vi "top_GameMode.vi"() -> ()   [LabVIEW 2014]
uses:
  <vilib>/sound2/lvsound2.llb/Sound Data Format.ctl
  <vilib>/sound2/lvsound2.llb/Sound Output Set Volume (Single).vi
  <vilib>/Utility/inputDevices.llb/keyboardAcquire.vi
  <vilib>/sound2/lvsound2.llb/Sound Output Write (DBL Single).vi
  <vilib>/Utility/inputDevices.llb/closeKeyboard.vi
  <vilib>/measure/NI_MABase.lvlib
panel:
  in  "stop":bool
  out "Your Score":dbl
  out "score":i32
  out "appended array 2":u32[](array[numeric])
  out "24":bool
  out "23":bool
  out "22":bool
  out "21":bool
  out "20":bool
  out "19":bool
  out "18":bool
  out "17":bool
  out "16":bool
  out "15":bool caption="Boolean 15"
  out "14":bool caption="Boolean 14"
  out "13":bool caption="Boolean 13"
  out "12":bool caption="Boolean 12"
  out "11":bool
  out "10":bool
  out "9":bool
  out "8":bool
  out "7":bool
  out "6":bool
  out "5":bool
  out "4":bool
  in  "Volume":dbl=70.0
  in  "Mode":enum16{"keypad", "button"}(ring)
  in  "Cluster":T1
  out "element 2":T2(ring)
  out "press time":u32[](array[numeric])
  out "String":string="3"
  out "3":bool
  out "2":bool
  out "1":bool
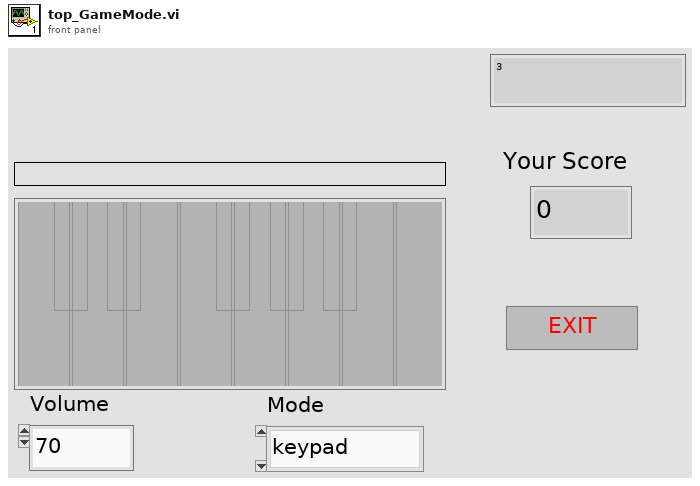
[diagram p1: front panel]
types:
  T1 = cluster{"c 2":bool, "c 3":bool, "c 4":bool, "c 5":bool, "c 6":bool, "c 7":bool, "c 8":bool, "c 9":bool, "c":bool, "c 10":bool, "c 11":bool, "c 12":bool, "c 13":bool}
  T2 = enum16{"0", "1", "2", "3", "4", "5", "6", "7", "8", "9", "A", "B", "C", "D", "E", "F", "G", "H", "I", "J", "K", "L", "M", "N", "O", "P", "Q", "R", "S", "T", "U", "V", "W", "X", "Y", "Z", "F1", "F2", "F3", "F4", "F5", "F6", "F7", "F8", "F9", "F10", "F11", "F12", "F13", "F14", "F15", "ADD", "BACK", "BACKSLASH", "CAPITAL", "COMMA", "DECIMAL", "DELETE", "DIVIDE", "DOWN", "END", "EQUALS", "ESCAPE", "GRAVE (`)", "HOME", "INSERT", "LBRACKET", "LCONTROL", "LEFT", "L ALT", "LSHIFT", "LWIN", "MINUS", "MULTIPLY", "NEXT", "NUMLOCK", "NUMPAD_0", "NUMPAD_1", "NUMPAD_2", "NUMPAD_3", "NUMPAD_4", "NUMPAD_5", "NUMPAD_6", "NUMPAD_7", "NUMPAD_8", "NUMPAD_9", "PAUSE", "PERIOD", "PRIOR (PG UP)", "RBRACKET", "RCONTROL", "RETURN", "RIGHT", "R ALT", "RSHIFT", "RWIN", "SCROLL", "SEMICOLON", "SLASH", "SPACE", "SUBTRACT", "TAB", "UP", "ENTER (num pad)", "' (quote)"}
  T3 = typedef "Sound Data Format.ctl" = cluster{"sample rate (S/s)":dbl, "number of channels":i32, "bits per sample":i32}
  T4 = typedef "Sound Output Task ID.ctl" = u32
  T5 = cluster{"sample rate (S/s)":dbl, "number of samples/ch":i32}
  T6 = enum16{"0", "1", "2", "3", "4", "5", "6", "7", "8", "9", "A", "B", "C", "D", "E", "F", "G", "H", "I", "J", "K", "L", "M", "N", "O", "P", "Q", "R", "S", "T", "U", "V", "W", "X", "Y", "Z", "F1", "F2", "F3", "F4", "F5", "F6", "F7", "F8", "F9", "F10", "F11", "F12", "F13", "F14", "F15", "ADD", "BACK", "BACKSLASH", "CAPITAL", "COMMA", "DECIMAL", "DELETE", "DIVIDE", "DOWN", "END", "EQUALS", "ESCAPE", "GRAVE (`)", "HOME", "INSERT", "LBRACKET", "LCONTROL", "LEFT", "L ALT", "LSHIFT", "LWIN", "MINUS", "MULTIPLY", "NEXT", "NUMLOCK", "NUMPAD_0", "NUMPAD_1", "NUMPAD_2", "NUMPAD_3", "NUMPAD_4", "NUMPAD_5", "NUMPAD_6", "NUMPAD_7", "NUMPAD_8", "NUMPAD_9", "PAUSE", "PERIOD", "PRIOR (PG UP)", "RBRACKET", "RCONTROL", "RETURN", "RIGHT", "R ALT", "RSHIFT", "RWIN", "SCROLL", "SEMICOLON", "SLASH", "SPACE", "SUBTRACT", "TAB", "UP", "ENTER (num pad)", "' (quote)"}[]
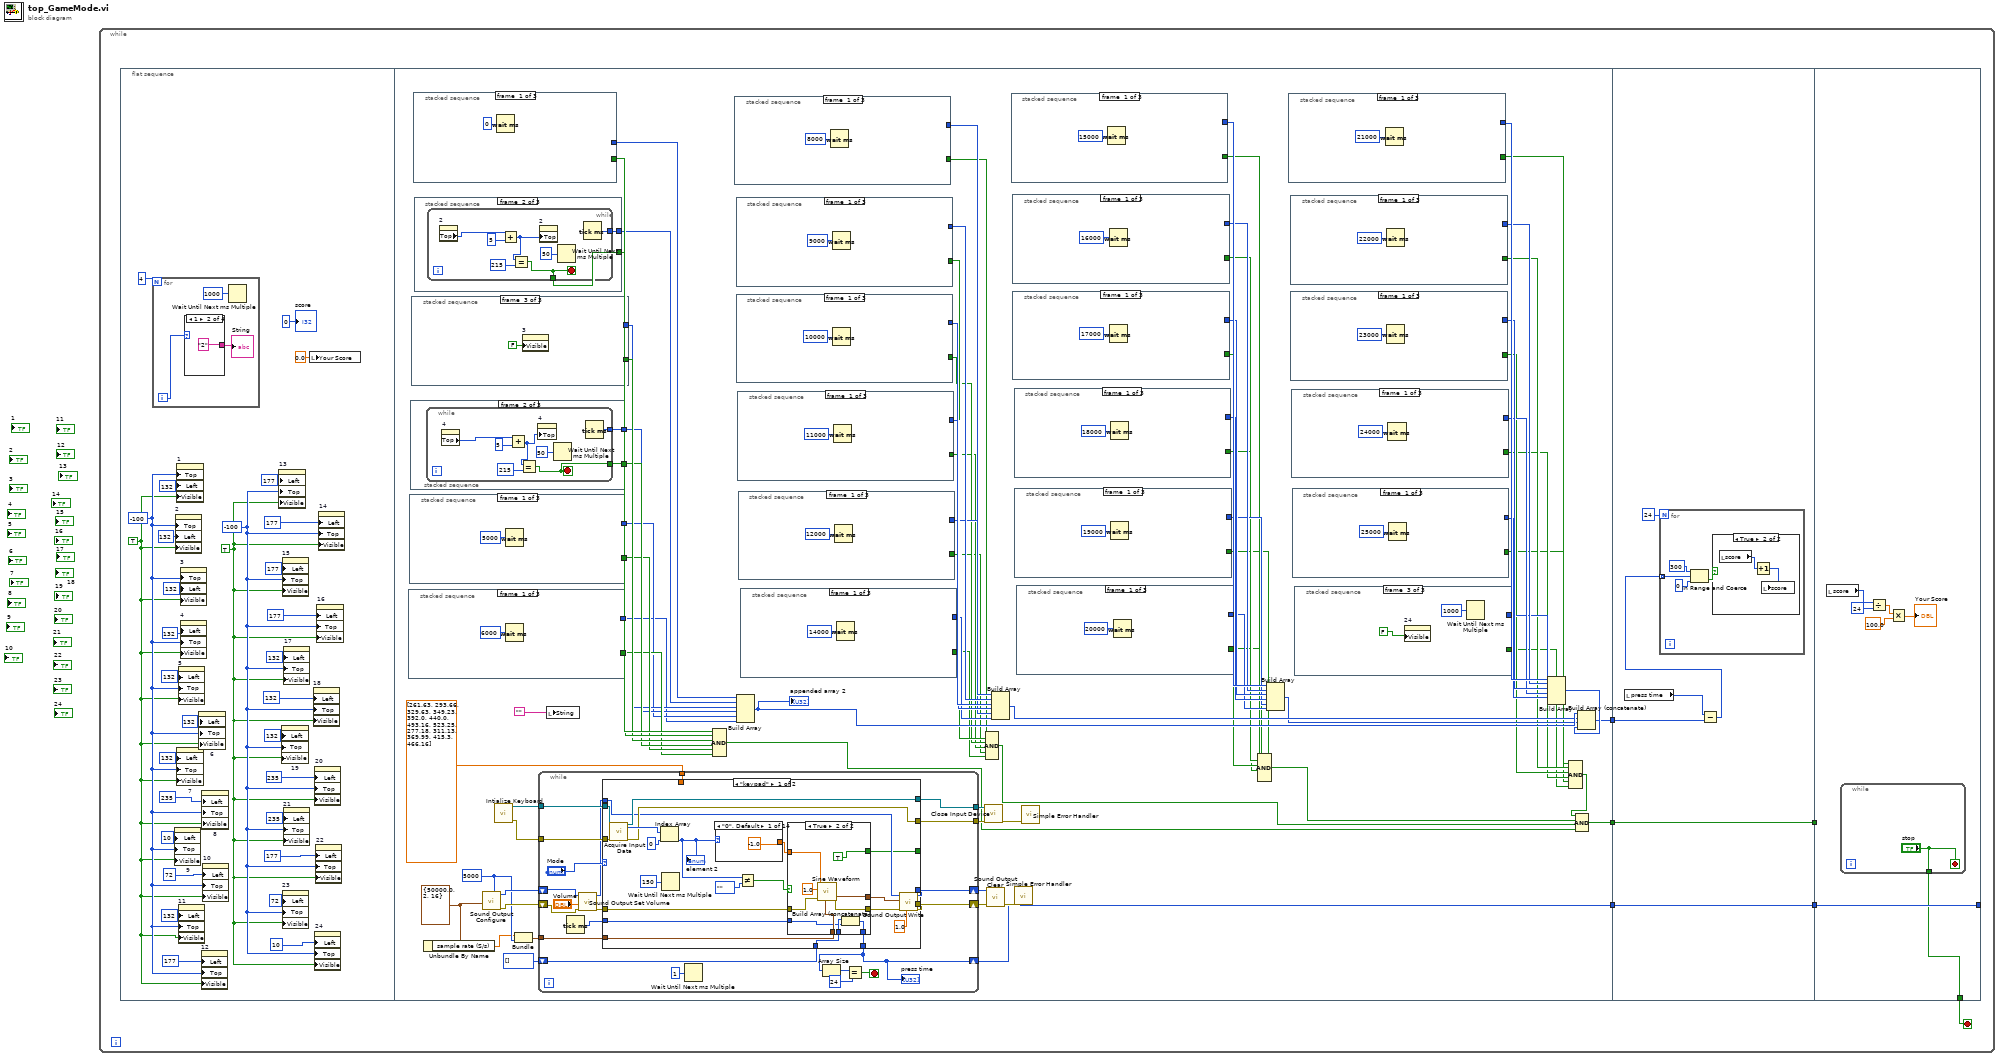
[diagram p0: block diagram]
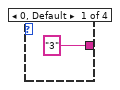
[diagram p2: hidden frame]
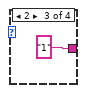
[diagram p3: hidden frame]
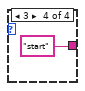
[diagram p4: hidden frame]
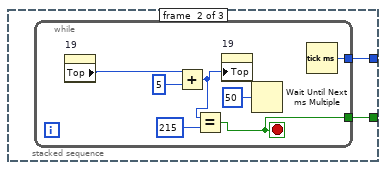
[diagram p5: hidden frame]
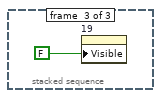
[diagram p6: hidden frame]
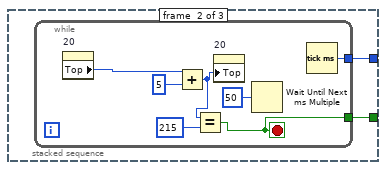
[diagram p7: hidden frame]
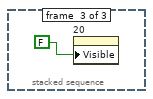
[diagram p8: hidden frame]
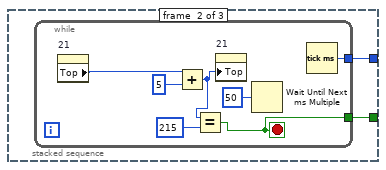
[diagram p9: hidden frame]
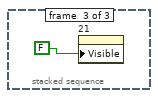
[diagram p10: hidden frame]
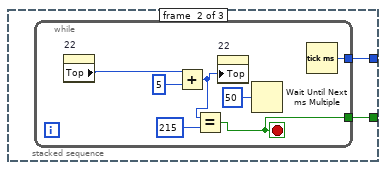
[diagram p11: hidden frame]
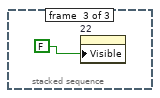
[diagram p12: hidden frame]
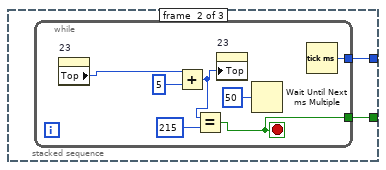
[diagram p13: hidden frame]
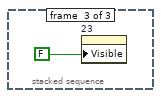
[diagram p14: hidden frame]
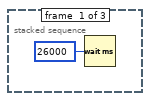
[diagram p15: hidden frame]
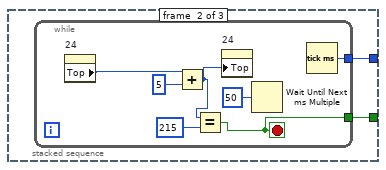
[diagram p16: hidden frame]
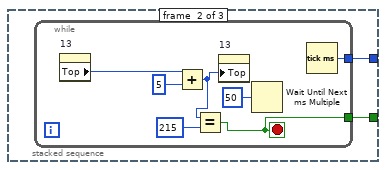
[diagram p17: hidden frame]
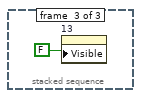
[diagram p18: hidden frame]
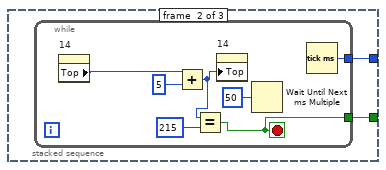
[diagram p19: hidden frame]
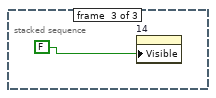
[diagram p20: hidden frame]
diagram:
  n1 = while {
    stop <- w1 stop-if-true
    n2 = flat-sequence {
      tunnel: [w104] -> w6
      tunnel: [w47] -> w5
      tunnel: [w46] -> w2
      tunnel: w6 -> [w496]
      tunnel: w5 -> [w495]
      tunnel: [w496] -> w4
      tunnel: [w491] -> w3
      tunnel: w2 -> [w491]
      tunnel: [w509] -> _
      tunnel: w4 -> [w509]
      tunnel: w3 -> [_]
      tunnel: [w503] -> w1
      frame #0 {
        w9 = TRUE
        w10 = TRUE
        w32 = -100
        w33 = -100
        n3 = for {
          N: 4 -> [_]
          i -> [w40]
          n4 = case shown="1" w40 {
            tunnel: ["3" "2" "1" "start"] -> w38
            frame 0, Default {
            }
            frame 1 {
            }
            frame 2 {
            }
            frame 3 {
            }
          }
          "String" <- w38
          n5 = Wait Until Next ms Multiple(millisecond multiple=u32 1000) -> ()  [unwired: 1 out]
        }
        n6 = property on="9" class="Bool (strict)"("Left"=10 ("Position:Left"), "Top"=w33, "Visible"=w10) -> ()  [unwired: 2 in, 2 out]
        n7 = property on="2" class="Bool (strict)"("Top"=w33, "Left"=132 ("Position:Left"), "Visible"=w10) -> ()  [unwired: 2 in, 2 out]
        n8 = property on="1" class="Bool (strict)"("Top"=w33, "Left"=132 ("Position:Left"), "Visible"=w10) -> ()  [unwired: 2 in, 2 out]
        n9 = property on="7" class="Bool (strict)"("Left"=132 ("Position:Left"), "Top"=w33, "Visible"=w10) -> ()  [unwired: 2 in, 2 out]
        n10 = property on="5" class="Bool (strict)"("Left"=132 ("Position:Left"), "Top"=w33, "Visible"=w10) -> ()  [unwired: 2 in, 2 out]
        n11 = property on="11" class="Bool (strict)"("Left"=132 ("Position:Left"), "Top"=w33, "Visible"=w10) -> ()  [unwired: 2 in, 2 out]
        n12 = property on="3" class="Bool (strict)"("Top"=w33, "Left"=132 ("Position:Left"), "Visible"=w10) -> ()  [unwired: 2 in, 2 out]
        n13 = property on="4" class="Bool (strict)"("Left"=132 ("Position:Left"), "Top"=w33, "Visible"=w10) -> ()  [unwired: 2 in, 2 out]
        n14 = property on="6" class="Bool (strict)"("Left"=132 ("Position:Left"), "Top"=w33, "Visible"=w10) -> ()  [unwired: 2 in, 2 out]
        n15 = property on="12" class="Bool (strict)"("Left"=177 ("Position:Left"), "Top"=w33, "Visible"=w10) -> ()  [unwired: 2 in, 2 out]
        n16 = property on="8" class="Bool (strict)"("Left"=235 ("Position:Left"), "Top"=w33, "Visible"=w10) -> ()  [unwired: 2 in, 2 out]
        n17 = property on="10" class="Bool (strict)"("Left"=72 ("Position:Left"), "Top"=w33, "Visible"=w10) -> ()  [unwired: 2 in, 2 out]
        n18 = property on="13" class="Bool (strict)"("Left"=177 ("Position:Left"), "Top"=w32, "Visible"=w9) -> ()  [unwired: 2 in, 2 out]
        n19 = property on="19" class="Bool (strict)"("Left"=132 ("Position:Left"), "Top"=w32, "Visible"=w9) -> ()  [unwired: 2 in, 2 out]
        n20 = property on="15" class="Bool (strict)"("Left"=177 ("Position:Left"), "Top"=w32, "Visible"=w9) -> ()  [unwired: 2 in, 2 out]
        n21 = property on="23" class="Bool (strict)"("Left"=72 ("Position:Left"), "Top"=w32, "Visible"=w9) -> ()  [unwired: 2 in, 2 out]
        n22 = property on="17" class="Bool (strict)"("Left"=132 ("Position:Left"), "Top"=w32, "Visible"=w9) -> ()  [unwired: 2 in, 2 out]
        n23 = property on="21" class="Bool (strict)"("Left"=235 ("Position:Left"), "Top"=w32, "Visible"=w9) -> ()  [unwired: 2 in, 2 out]
        n24 = local write "Your Score"(0.0 ("your score")) -> ()
        n25 = property on="18" class="Bool (strict)"("Left"=132 ("Position:Left"), "Top"=w32, "Visible"=w9) -> ()  [unwired: 2 in, 2 out]
        n26 = property on="20" class="Bool (strict)"("Left"=235 ("Position:Left"), "Top"=w32, "Visible"=w9) -> ()  [unwired: 2 in, 2 out]
        n27 = property on="24" class="Bool (strict)"("Left"=10 ("Position:Left"), "Top"=w32, "Visible"=w9) -> ()  [unwired: 2 in, 2 out]
        n28 = property on="22" class="Bool (strict)"("Left"=177 ("Position:Left"), "Top"=w32, "Visible"=w9) -> ()  [unwired: 2 in, 2 out]
        n29 = property on="16" class="Bool (strict)"("Left"=177 ("Position:Left"), "Top"=w32, "Visible"=w9) -> ()  [unwired: 2 in, 2 out]
        n30 = property on="14" class="Bool (strict)"("Left"=177 ("Position:Left"), "Top"=w32, "Visible"=w9) -> ()  [unwired: 2 in, 2 out]
        "score" <- 0
      }
      frame #1 {
        w117 = 5000 ("number of samples/ch")
        w118 = T3 {"sample rate (S/s)"=50000.0, "number of channels"=2, "bits per sample"=16} ("sound format")
        n31 = stacked-sequence {
          tunnel: [_ w333 _] -> w98
          tunnel: [_ w332 _] -> w92
          frame #0 {
            n32 = Wait (ms)(milliseconds to wait=u32 6000) -> ()  [unwired: 1 out]
          }
          frame #1 {
            n33 = while {
              tunnel: [w337] -> w333
              tunnel: [w336] -> w332
              stop <- w337 stop-if-true
              n34 = property on="6" class="Bool (strict)"() -> ("Top"=w334:i32)  [unwired: 2 in, 2 out]
              n35 = Add(x=w334, y=5) -> (x+y=w335:i32)
              n36 = Equal?(x=w335, y=215) -> (x = y?=w337:bool)
              n37 = property on="6" class="Bool (strict)"("Top"=w335) -> ()  [unwired: 2 in, 2 out]
              n38 = Wait Until Next ms Multiple(millisecond multiple=u32 50) -> ()  [unwired: 1 out]
              n39 = Tick Count (ms)() -> (millisecond timer value=w336:u32)
            }
          }
          frame #2 {
            n40 = property on="6" class="Bool (strict)"("Visible"=FALSE) -> ()  [unwired: 2 in, 2 out]
          }
        }
        n41 = stacked-sequence {
          tunnel: [_ w344 _] -> w99
          tunnel: [_ w343 _] -> w93
          frame #0 {
            n42 = Wait (ms)(milliseconds to wait=u32 5000) -> ()  [unwired: 1 out]
          }
          frame #1 {
            n43 = while {
              tunnel: [w348] -> w344
              tunnel: [w347] -> w343
              stop <- w348 stop-if-true
              n44 = property on="5" class="Bool (strict)"() -> ("Top"=w345:i32)  [unwired: 2 in, 2 out]
              n45 = Add(x=w345, y=5) -> (x+y=w346:i32)
              n46 = Equal?(x=w346, y=215) -> (x = y?=w348:bool)
              n47 = property on="5" class="Bool (strict)"("Top"=w346) -> ()  [unwired: 2 in, 2 out]
              n48 = Wait Until Next ms Multiple(millisecond multiple=u32 50) -> ()  [unwired: 1 out]
              n49 = Tick Count (ms)() -> (millisecond timer value=w347:u32)
            }
          }
          frame #2 {
            n50 = property on="5" class="Bool (strict)"("Visible"=FALSE) -> ()  [unwired: 2 in, 2 out]
          }
        }
        n51 = stacked-sequence {
          tunnel: [_ w355 _] -> w100
          tunnel: [_ w354 _] -> w94
          frame #0 {
            n52 = Wait (ms)(milliseconds to wait=u32 4000) -> ()  [unwired: 1 out]
          }
          frame #1 {
            n53 = while {
              tunnel: [w359] -> w355
              tunnel: [w358] -> w354
              stop <- w359 stop-if-true
              n54 = property on="4" class="Bool (strict)"() -> ("Top"=w356:i32)  [unwired: 2 in, 2 out]
              n55 = Add(x=w356, y=5) -> (x+y=w357:i32)
              n56 = Equal?(x=w357, y=215) -> (x = y?=w359:bool)
              n57 = property on="4" class="Bool (strict)"("Top"=w357) -> ()  [unwired: 2 in, 2 out]
              n58 = Wait Until Next ms Multiple(millisecond multiple=u32 50) -> ()  [unwired: 1 out]
              n59 = Tick Count (ms)() -> (millisecond timer value=w358:u32)
            }
          }
          frame #2 {
            n60 = property on="4" class="Bool (strict)"("Visible"=FALSE) -> ()  [unwired: 2 in, 2 out]
          }
        }
        n61 = stacked-sequence {
          tunnel: [_ w471 _] -> w101
          tunnel: [_ w470 _] -> w95
          frame #0 {
            n62 = Wait (ms)(milliseconds to wait=u32 2000) -> ()  [unwired: 1 out]
          }
          frame #1 {
            n63 = while {
              tunnel: [w474] -> w471
              tunnel: [w472] -> w470
              stop <- w474 stop-if-true
              n64 = property on="3" class="Bool (strict)"() -> ("Top"=w475:i32)  [unwired: 2 in, 2 out]
              n65 = Add(x=w475, y=5) -> (x+y=w473:i32)
              n66 = Equal?(x=w473, y=215) -> (x = y?=w474:bool)
              n67 = property on="3" class="Bool (strict)"("Top"=w473) -> ()  [unwired: 2 in, 2 out]
              n68 = Wait Until Next ms Multiple(millisecond multiple=u32 50) -> ()  [unwired: 1 out]
              n69 = Tick Count (ms)() -> (millisecond timer value=w472:u32)
            }
          }
          frame #2 {
            n70 = property on="3" class="Bool (strict)"("Visible"=FALSE) -> ()  [unwired: 2 in, 2 out]
          }
        }
        n71 = stacked-sequence {
          tunnel: [_ w322 _] -> w103
          tunnel: [_ w321 _] -> w97
          frame #0 {
            n72 = Wait (ms)(milliseconds to wait=u32 0) -> ()  [unwired: 1 out]
          }
          frame #1 {
            n73 = while {
              tunnel: [w324] -> w322
              tunnel: [w323] -> w321
              stop <- w324 stop-if-true
              n74 = property on="1" class="Bool (strict)"() -> ("Top"=w328:i32)  [unwired: 2 in, 2 out]
              n75 = Add(x=w328, y=5) -> (x+y=w326:i32)
              n76 = Equal?(x=w326, y=215) -> (x = y?=w324:bool)
              n77 = property on="1" class="Bool (strict)"("Top"=w326) -> ()  [unwired: 2 in, 2 out]
              n78 = Wait Until Next ms Multiple(millisecond multiple=u32 50) -> ()  [unwired: 1 out]
              n79 = Tick Count (ms)() -> (millisecond timer value=w323:u32)
            }
          }
          frame #2 {
            n80 = property on="1" class="Bool (strict)"("Visible"=FALSE) -> ()  [unwired: 2 in, 2 out]
          }
        }
        n81 = stacked-sequence {
          tunnel: [_ w482 _] -> w102
          tunnel: [_ w481 _] -> w96
          frame #0 {
            n82 = Wait (ms)(milliseconds to wait=u32 1000) -> ()  [unwired: 1 out]
          }
          frame #1 {
            n83 = while {
              tunnel: [w484] -> w482
              tunnel: [w483] -> w481
              stop <- w484 stop-if-true
              n84 = property on="2" class="Bool (strict)"() -> ("Top"=w487:i32)  [unwired: 2 in, 2 out]
              n85 = Add(x=w487, y=5) -> (x+y=w485:i32)
              n86 = Equal?(x=w485, y=215) -> (x = y?=w484:bool)
              n87 = property on="2" class="Bool (strict)"("Top"=w485) -> ()  [unwired: 2 in, 2 out]
              n88 = Wait Until Next ms Multiple(millisecond multiple=u32 50) -> ()  [unwired: 1 out]
              n89 = Tick Count (ms)() -> (millisecond timer value=w483:u32)
            }
          }
          frame #2 {
            n90 = property on="2" class="Bool (strict)"("Visible"=FALSE) -> ()  [unwired: 2 in, 2 out]
          }
        }
        n91 = Unbundle By Name(w118) -> ("sample rate (S/s)"=w116:dbl)
        n92 = call <vilib>:"Sound Output Configure.vi"("number of samples/ch"=w117, "sound format"=w118) -> ("error out"=w119:errorcluster, "task ID"=w120:T4)  [unwired: 8 in]
        n93 = call <vilib>:"Intialize Keyboard.vi"() -> ("error out"=w109:errorcluster, "device ID"=w108:refnum<k1>)  [unwired: 10 in]
        n94 = Bundle("sample rate (S/s)"=w116, "number of samples/ch"=w117) -> (w115:T5)  [unwired: 1 in]
        n95 = while {
          tunnel: w115 -> [w381]
          tunnel: dbl[] [261.63, 293.66, 329.63, 349.23, 392.0, 440.0, 493.16, 523.25, 277.18, 311.13, 369.99, 415.3, 466.16] -> [w377]
          shift-right: [w380] -> w114
          shift-left: w120 -> [w383]
          shift-right: [w379] -> w113
          shift-left: w119 -> [w378]
          tunnel: w109 -> [w374]
          tunnel: w108 -> [w373]
          tunnel: [w372] -> w107
          tunnel: [w371] -> w106
          shift-right: [w367] -> w104
          shift-left: u32[] [] -> [w369]
          stop <- w364 stop-if-true
          n96 = Tick Count (ms)() -> (millisecond timer value=w368:u32)
          n97 = call-poly <vilib>:"Sound Output Set Volume.vi"("error in (no error)"=w378, "volume"="Volume", "task ID"=w383) -> ("error out"=w382:errorcluster, "task ID out"=w370:T4)  [unwired: 7 in]
          n98 = case shown="\"keypad\"" "Mode" {
            tunnel: w382 -> [w394 w453]
            tunnel: w381 -> [w393 w450]
            tunnel: w370 -> [w392 w449]
            tunnel: [w391 w448] -> w380
            tunnel: [w390 w447] -> w379
            tunnel: w377 -> [_ w446]
            tunnel: w374 -> [w398 _]
            tunnel: w373 -> [w397 _]
            tunnel: [w396 _] -> w372
            tunnel: [w395 _] -> w371
            tunnel: [w389 w438] -> _
            tunnel: w369 -> [w388 w437]
            tunnel: [w387 w436] -> w367
            tunnel: w368 -> [w386 w435]
            frame "keypad" {
              n99 = call-poly <vilib>:"Acquire Input Data.vi"("device ID"=w397, "error in (no error)"=w398) -> ("device ID"=w396:refnum<k1>, "keys pressed"=w403:T6, "error out"=w395:errorcluster)  [unwired: 15 in]
              n100 = Index Array(array=w403, index=0) -> (element=w407:T2)
              "element 2" <- w407
              n101 = Wait Until Next ms Multiple(millisecond multiple=u32 150) -> ()  [unwired: 1 out]
              n102 = case shown="\"0\", Default" w407 {
                tunnel: [-1.0 261.63 277.18 293.66 311.13 329.63 349.23 369.99 392 415.3 440 466.16 493.88 523.25] -> w402
                frame "0", Default {
                }
                frame "S" {
                }
                frame "E" {
                }
                frame "D" {
                }
                frame "R" {
                }
                frame "F" {
                }
                frame "G" {
                }
                frame "Y" {
                }
                frame "H" {
                }
                frame "U" {
                }
                frame "J" {
                }
                frame "I" {
                }
                frame "K" {
                }
                frame "L" {
                }
              }
              n103 = Not Equal?(x=w407, y=enum16{""}."") -> (x != y?=w406:bool)
              n104 = case shown="True" w406 {
                tunnel: w394 -> [w410 w419]
                tunnel: [_ w418] -> w399
                tunnel: [w410 w417] -> w400
                tunnel: w393 -> [_ w416]
                tunnel: w402 -> [_ w415]
                tunnel: [FALSE TRUE] -> w389
                tunnel: w388 -> [w408 w413]
                tunnel: [w408 w412] -> w387
                tunnel: w386 -> [_ w411]
                frame False {
                }
                frame True {
                  n105 = call <vilib>:"Sine Waveform.vi"("sampling info"=w416, "error in (no error)"=w419, "amplitude"=1.0, "frequency"=w415) -> ("error out"=w417:errorcluster, "signal out"=w418:waveform(dbl))  [unwired: 6 in]
                  n106 = Build Array (concatenate)(w413, w411) -> (w412:u32[])
                }
              }
              n107 = call-poly <vilib>:"Sound Output Write.vi"("timeout (sec)"=1.0, "error in (no error)"=w400, "data"=w399, "task ID"=w392) -> ("error out"=w390:errorcluster, "task ID out"=w391:T4)  [unwired: 6 in]
            }
            frame "button", Default {
              n108 = Cluster To Array(cluster="Cluster") -> (array=w441:bool[])
              n109 = Or Array Elements(Boolean array=w441) -> (logical OR=w440:bool)
              n110 = Search 1D Array(1D array=w441, element=TRUE, start index (0)=0) -> (index of element=w439:i32)
              n111 = case shown="True" w440 {
                tunnel: w453 -> [w456 w467]
                tunnel: [_ w466] -> w452
                tunnel: [w456 w465] -> w451
                tunnel: w450 -> [_ w464]
                tunnel: w446 -> [_ w463]
                tunnel: w439 -> [_ w462]
                tunnel: [FALSE TRUE] -> w438
                tunnel: w437 -> [w454 w459]
                tunnel: [w454 w458] -> w436
                tunnel: w435 -> [_ w457]
                frame False {
                }
                frame True {
                  n112 = Index Array(array=w463, index=w462) -> (element=w461:dbl)
                  n113 = call <vilib>:"Sine Waveform.vi"("sampling info"=w464, "error in (no error)"=w467, "amplitude"=1.0, "frequency"=w461) -> ("error out"=w465:errorcluster, "signal out"=w466:waveform(dbl))  [unwired: 6 in]
                  n114 = Build Array (concatenate)(w459, w457) -> (w458:u32[])
                }
              }
              n115 = call-poly <vilib>:"Sound Output Write.vi"("timeout (sec)"=1.0, "error in (no error)"=w451, "data"=w452, "task ID"=w449) -> ("error out"=w447:errorcluster, "task ID out"=w448:T4)  [unwired: 6 in]
            }
          }
          "press time" <- w367
          n116 = Wait Until Next ms Multiple(millisecond multiple=u32 1) -> ()  [unwired: 1 out]
          n117 = Array Size(array=w367) -> (size(s)=w366:i32)
          n118 = Equal?(x=w366, y=24) -> (x = y?=w364:bool)
        }
        n119 = local write "String"("") -> ()
        n120 = Compound Arithmetic op=AND(w103, w102, w101, w100, w99, w98) -> (w48:bool)
        n121 = stacked-sequence {
          tunnel: [_ w256 _] -> w69
          tunnel: [_ w255 _] -> w91
          frame #0 {
            n122 = Wait (ms)(milliseconds to wait=u32 8000) -> ()  [unwired: 1 out]
          }
          frame #1 {
            n123 = while {
              tunnel: [w260] -> w256
              tunnel: [w259] -> w255
              stop <- w260 stop-if-true
              n124 = property on="7" class="Bool (strict)"() -> ("Top"=w258:i32)  [unwired: 2 in, 2 out]
              n125 = Add(x=w258, y=5) -> (x+y=w257:i32)
              n126 = Equal?(x=w257, y=215) -> (x = y?=w260:bool)
              n127 = property on="7" class="Bool (strict)"("Top"=w257) -> ()  [unwired: 2 in, 2 out]
              n128 = Wait Until Next ms Multiple(millisecond multiple=u32 50) -> ()  [unwired: 1 out]
              n129 = Tick Count (ms)() -> (millisecond timer value=w259:u32)
            }
          }
          frame #2 {
            n130 = property on="7" class="Bool (strict)"("Visible"=FALSE) -> ()  [unwired: 2 in, 2 out]
          }
        }
        n131 = stacked-sequence {
          tunnel: [_ w267 _] -> w68
          tunnel: [_ w266 _] -> w90
          frame #0 {
            n132 = Wait (ms)(milliseconds to wait=u32 9000) -> ()  [unwired: 1 out]
          }
          frame #1 {
            n133 = while {
              tunnel: [w271] -> w267
              tunnel: [w270] -> w266
              stop <- w271 stop-if-true
              n134 = property on="8" class="Bool (strict)"() -> ("Top"=w268:i32)  [unwired: 2 in, 2 out]
              n135 = Add(x=w268, y=5) -> (x+y=w269:i32)
              n136 = Equal?(x=w269, y=215) -> (x = y?=w271:bool)
              n137 = property on="8" class="Bool (strict)"("Top"=w269) -> ()  [unwired: 2 in, 2 out]
              n138 = Wait Until Next ms Multiple(millisecond multiple=u32 50) -> ()  [unwired: 1 out]
              n139 = Tick Count (ms)() -> (millisecond timer value=w270:u32)
            }
          }
          frame #2 {
            n140 = property on="8" class="Bool (strict)"("Visible"=FALSE) -> ()  [unwired: 2 in, 2 out]
          }
        }
        n141 = stacked-sequence {
          tunnel: [_ w278 _] -> w67
          tunnel: [_ w277 _] -> w89
          frame #0 {
            n142 = Wait (ms)(milliseconds to wait=u32 10000) -> ()  [unwired: 1 out]
          }
          frame #1 {
            n143 = while {
              tunnel: [w282] -> w278
              tunnel: [w281] -> w277
              stop <- w282 stop-if-true
              n144 = property on="9" class="Bool (strict)"() -> ("Top"=w280:i32)  [unwired: 2 in, 2 out]
              n145 = Add(x=w280, y=5) -> (x+y=w279:i32)
              n146 = Equal?(x=w279, y=215) -> (x = y?=w282:bool)
              n147 = property on="9" class="Bool (strict)"("Top"=w279) -> ()  [unwired: 2 in, 2 out]
              n148 = Wait Until Next ms Multiple(millisecond multiple=u32 50) -> ()  [unwired: 1 out]
              n149 = Tick Count (ms)() -> (millisecond timer value=w281:u32)
            }
          }
          frame #2 {
            n150 = property on="9" class="Bool (strict)"("Visible"=FALSE) -> ()  [unwired: 2 in, 2 out]
          }
        }
        n151 = Build Array(w97, w96, w95, w94, w93, w92) -> (w73:u32[])
        "appended array 2" <- w73
        n152 = stacked-sequence {
          tunnel: [_ w289 _] -> w66
          tunnel: [_ w288 _] -> w88
          frame #0 {
            n153 = Wait (ms)(milliseconds to wait=u32 11000) -> ()  [unwired: 1 out]
          }
          frame #1 {
            n154 = while {
              tunnel: [w293] -> w289
              tunnel: [w292] -> w288
              stop <- w293 stop-if-true
              n155 = property on="10" class="Bool (strict)"() -> ("Top"=w291:i32)  [unwired: 2 in, 2 out]
              n156 = Add(x=w291, y=5) -> (x+y=w290:i32)
              n157 = Equal?(x=w290, y=215) -> (x = y?=w293:bool)
              n158 = property on="10" class="Bool (strict)"("Top"=w290) -> ()  [unwired: 2 in, 2 out]
              n159 = Wait Until Next ms Multiple(millisecond multiple=u32 50) -> ()  [unwired: 1 out]
              n160 = Tick Count (ms)() -> (millisecond timer value=w292:u32)
            }
          }
          frame #2 {
            n161 = property on="10" class="Bool (strict)"("Visible"=FALSE) -> ()  [unwired: 2 in, 2 out]
          }
        }
        n162 = stacked-sequence {
          tunnel: [_ w300 _] -> w65
          tunnel: [_ w299 _] -> w87
          frame #0 {
            n163 = Wait (ms)(milliseconds to wait=u32 12000) -> ()  [unwired: 1 out]
          }
          frame #1 {
            n164 = while {
              tunnel: [w304] -> w300
              tunnel: [w303] -> w299
              stop <- w304 stop-if-true
              n165 = property on="11" class="Bool (strict)"() -> ("Top"=w302:i32)  [unwired: 2 in, 2 out]
              n166 = Add(x=w302, y=5) -> (x+y=w301:i32)
              n167 = Equal?(x=w301, y=215) -> (x = y?=w304:bool)
              n168 = property on="11" class="Bool (strict)"("Top"=w301) -> ()  [unwired: 2 in, 2 out]
              n169 = Wait Until Next ms Multiple(millisecond multiple=u32 50) -> ()  [unwired: 1 out]
              n170 = Tick Count (ms)() -> (millisecond timer value=w303:u32)
            }
          }
          frame #2 {
            n171 = property on="11" class="Bool (strict)"("Visible"=FALSE) -> ()  [unwired: 2 in, 2 out]
          }
        }
        n172 = stacked-sequence {
          tunnel: [_ w311 _] -> w64
          tunnel: [_ w310 _] -> w86
          frame #0 {
            n173 = Wait (ms)(milliseconds to wait=u32 14000) -> ()  [unwired: 1 out]
          }
          frame #1 {
            n174 = while {
              tunnel: [w315] -> w311
              tunnel: [w314] -> w310
              stop <- w315 stop-if-true
              n175 = property on="12" class="Bool (strict)"() -> ("Top"=w313:i32)  [unwired: 2 in, 2 out]
              n176 = Add(x=w313, y=5) -> (x+y=w312:i32)
              n177 = Equal?(x=w312, y=215) -> (x = y?=w315:bool)
              n178 = property on="12" class="Bool (strict)"("Top"=w312) -> ()  [unwired: 2 in, 2 out]
              n179 = Wait Until Next ms Multiple(millisecond multiple=u32 50) -> ()  [unwired: 1 out]
              n180 = Tick Count (ms)() -> (millisecond timer value=w314:u32)
            }
          }
          frame #2 {
            n181 = property on="12" class="Bool (strict)"("Visible"=FALSE) -> ()  [unwired: 2 in, 2 out]
          }
        }
        n182 = call-poly <vilib>:"Close Input Device.vi"("error in (no error)"=w106, "device ID"=w107) -> ("error out"=w110:errorcluster)  [unwired: 8 in]
        n183 = Compound Arithmetic op=AND(w69, w68, w67, w66, w65, w64) -> (w49:bool)
        n184 = call <vilib>:"Sound Output Clear.vi"("error in (no error)"=w113, "task ID"=w114) -> ("error out"=w112:errorcluster)  [unwired: 9 in]
        n185 = Build Array(w91, w90, w89, w88, w87, w86) -> (w72:u32[])
        n186 = stacked-sequence {
          tunnel: [_ w190 _] -> w63
          tunnel: [_ w189 _] -> w85
          frame #0 {
            n187 = Wait (ms)(milliseconds to wait=u32 15000) -> ()  [unwired: 1 out]
          }
          frame #1 {
            n188 = while {
              tunnel: [w194] -> w190
              tunnel: [w193] -> w189
              stop <- w194 stop-if-true
              n189 = property on="13" class="Bool (strict)"() -> ("Top"=w192:i32)  [unwired: 2 in, 2 out]
              n190 = Add(x=w192, y=5) -> (x+y=w191:i32)
              n191 = Equal?(x=w191, y=215) -> (x = y?=w194:bool)
              n192 = property on="13" class="Bool (strict)"("Top"=w191) -> ()  [unwired: 2 in, 2 out]
              n193 = Wait Until Next ms Multiple(millisecond multiple=u32 50) -> ()  [unwired: 1 out]
              n194 = Tick Count (ms)() -> (millisecond timer value=w193:u32)
            }
          }
          frame #2 {
            n195 = property on="13" class="Bool (strict)"("Visible"=FALSE) -> ()  [unwired: 2 in, 2 out]
          }
        }
        n196 = stacked-sequence {
          tunnel: [_ w201 _] -> w62
          tunnel: [_ w200 _] -> w84
          frame #0 {
            n197 = Wait (ms)(milliseconds to wait=u32 16000) -> ()  [unwired: 1 out]
          }
          frame #1 {
            n198 = while {
              tunnel: [w205] -> w201
              tunnel: [w204] -> w200
              stop <- w205 stop-if-true
              n199 = property on="14" class="Bool (strict)"() -> ("Top"=w203:i32)  [unwired: 2 in, 2 out]
              n200 = Add(x=w203, y=5) -> (x+y=w202:i32)
              n201 = Equal?(x=w202, y=215) -> (x = y?=w205:bool)
              n202 = property on="14" class="Bool (strict)"("Top"=w202) -> ()  [unwired: 2 in, 2 out]
              n203 = Wait Until Next ms Multiple(millisecond multiple=u32 50) -> ()  [unwired: 1 out]
              n204 = Tick Count (ms)() -> (millisecond timer value=w204:u32)
            }
          }
          frame #2 {
            n205 = property on="14" class="Bool (strict)"("Visible"=FALSE) -> ()  [unwired: 2 in, 2 out]
          }
        }
        n206 = stacked-sequence {
          tunnel: [_ w212 _] -> w61
          tunnel: [_ w211 _] -> w83
          frame #0 {
            n207 = Wait (ms)(milliseconds to wait=u32 17000) -> ()  [unwired: 1 out]
          }
          frame #1 {
            n208 = while {
              tunnel: [w216] -> w212
              tunnel: [w215] -> w211
              stop <- w216 stop-if-true
              n209 = property on="15" class="Bool (strict)"() -> ("Top"=w214:i32)  [unwired: 2 in, 2 out]
              n210 = Add(x=w214, y=5) -> (x+y=w213:i32)
              n211 = Equal?(x=w213, y=215) -> (x = y?=w216:bool)
              n212 = property on="15" class="Bool (strict)"("Top"=w213) -> ()  [unwired: 2 in, 2 out]
              n213 = Wait Until Next ms Multiple(millisecond multiple=u32 50) -> ()  [unwired: 1 out]
              n214 = Tick Count (ms)() -> (millisecond timer value=w215:u32)
            }
          }
          frame #2 {
            n215 = property on="15" class="Bool (strict)"("Visible"=FALSE) -> ()  [unwired: 2 in, 2 out]
          }
        }
        n216 = stacked-sequence {
          tunnel: [_ w223 _] -> w60
          tunnel: [_ w222 _] -> w82
          frame #0 {
            n217 = Wait (ms)(milliseconds to wait=u32 18000) -> ()  [unwired: 1 out]
          }
          frame #1 {
            n218 = while {
              tunnel: [w227] -> w223
              tunnel: [w226] -> w222
              stop <- w227 stop-if-true
              n219 = property on="16" class="Bool (strict)"() -> ("Top"=w225:i32)  [unwired: 2 in, 2 out]
              n220 = Add(x=w225, y=5) -> (x+y=w224:i32)
              n221 = Equal?(x=w224, y=215) -> (x = y?=w227:bool)
              n222 = property on="16" class="Bool (strict)"("Top"=w224) -> ()  [unwired: 2 in, 2 out]
              n223 = Wait Until Next ms Multiple(millisecond multiple=u32 50) -> ()  [unwired: 1 out]
              n224 = Tick Count (ms)() -> (millisecond timer value=w226:u32)
            }
          }
          frame #2 {
            n225 = property on="16" class="Bool (strict)"("Visible"=FALSE) -> ()  [unwired: 2 in, 2 out]
          }
        }
        n226 = stacked-sequence {
          tunnel: [_ w234 _] -> w59
          tunnel: [_ w233 _] -> w81
          frame #0 {
            n227 = Wait (ms)(milliseconds to wait=u32 19000) -> ()  [unwired: 1 out]
          }
          frame #1 {
            n228 = while {
              tunnel: [w238] -> w234
              tunnel: [w237] -> w233
              stop <- w238 stop-if-true
              n229 = property on="17" class="Bool (strict)"() -> ("Top"=w236:i32)  [unwired: 2 in, 2 out]
              n230 = Add(x=w236, y=5) -> (x+y=w235:i32)
              n231 = Equal?(x=w235, y=215) -> (x = y?=w238:bool)
              n232 = property on="17" class="Bool (strict)"("Top"=w235) -> ()  [unwired: 2 in, 2 out]
              n233 = Wait Until Next ms Multiple(millisecond multiple=u32 50) -> ()  [unwired: 1 out]
              n234 = Tick Count (ms)() -> (millisecond timer value=w237:u32)
            }
          }
          frame #2 {
            n235 = property on="17" class="Bool (strict)"("Visible"=FALSE) -> ()  [unwired: 2 in, 2 out]
          }
        }
        n236 = call <vilib>:"Simple Error Handler.vi"("error in (no error)"=w112) -> ()  [unwired: 4 in, 5 out]
        n237 = stacked-sequence {
          tunnel: [_ w245 _] -> w58
          tunnel: [_ w244 _] -> w80
          frame #0 {
            n238 = Wait (ms)(milliseconds to wait=u32 20000) -> ()  [unwired: 1 out]
          }
          frame #1 {
            n239 = while {
              tunnel: [w249] -> w245
              tunnel: [w248] -> w244
              stop <- w249 stop-if-true
              n240 = property on="18" class="Bool (strict)"() -> ("Top"=w247:i32)  [unwired: 2 in, 2 out]
              n241 = Add(x=w247, y=5) -> (x+y=w246:i32)
              n242 = Equal?(x=w246, y=215) -> (x = y?=w249:bool)
              n243 = property on="18" class="Bool (strict)"("Top"=w246) -> ()  [unwired: 2 in, 2 out]
              n244 = Wait Until Next ms Multiple(millisecond multiple=u32 50) -> ()  [unwired: 1 out]
              n245 = Tick Count (ms)() -> (millisecond timer value=w248:u32)
            }
          }
          frame #2 {
            n246 = property on="18" class="Bool (strict)"("Visible"=FALSE) -> ()  [unwired: 2 in, 2 out]
          }
        }
        n247 = call <vilib>:"Simple Error Handler.vi"("error in (no error)"=w110) -> ()  [unwired: 4 in, 5 out]
        n248 = Compound Arithmetic op=AND(w63, w62, w61, w60, w59, w58) -> (w50:bool)
        n249 = Build Array(w85, w84, w83, w82, w81, w80) -> (w71:u32[])
        n250 = stacked-sequence {
          tunnel: [_ w123 _] -> w57
          tunnel: [_ w122 _] -> w79
          frame #0 {
            n251 = Wait (ms)(milliseconds to wait=u32 21000) -> ()  [unwired: 1 out]
          }
          frame #1 {
            n252 = while {
              tunnel: [w127] -> w123
              tunnel: [w126] -> w122
              stop <- w127 stop-if-true
              n253 = property on="19" class="Bool (strict)"() -> ("Top"=w125:i32)  [unwired: 2 in, 2 out]
              n254 = Add(x=w125, y=5) -> (x+y=w124:i32)
              n255 = Equal?(x=w124, y=215) -> (x = y?=w127:bool)
              n256 = property on="19" class="Bool (strict)"("Top"=w124) -> ()  [unwired: 2 in, 2 out]
              n257 = Wait Until Next ms Multiple(millisecond multiple=u32 50) -> ()  [unwired: 1 out]
              n258 = Tick Count (ms)() -> (millisecond timer value=w126:u32)
            }
          }
          frame #2 {
            n259 = property on="19" class="Bool (strict)"("Visible"=FALSE) -> ()  [unwired: 2 in, 2 out]
          }
        }
        n260 = stacked-sequence {
          tunnel: [_ w134 _] -> w56
          tunnel: [_ w133 _] -> w78
          frame #0 {
            n261 = Wait (ms)(milliseconds to wait=u32 22000) -> ()  [unwired: 1 out]
          }
          frame #1 {
            n262 = while {
              tunnel: [w138] -> w134
              tunnel: [w137] -> w133
              stop <- w138 stop-if-true
              n263 = property on="20" class="Bool (strict)"() -> ("Top"=w136:i32)  [unwired: 2 in, 2 out]
              n264 = Add(x=w136, y=5) -> (x+y=w135:i32)
              n265 = Equal?(x=w135, y=215) -> (x = y?=w138:bool)
              n266 = property on="20" class="Bool (strict)"("Top"=w135) -> ()  [unwired: 2 in, 2 out]
              n267 = Wait Until Next ms Multiple(millisecond multiple=u32 50) -> ()  [unwired: 1 out]
              n268 = Tick Count (ms)() -> (millisecond timer value=w137:u32)
            }
          }
          frame #2 {
            n269 = property on="20" class="Bool (strict)"("Visible"=FALSE) -> ()  [unwired: 2 in, 2 out]
          }
        }
        n270 = stacked-sequence {
          tunnel: [_ w145 _] -> w55
          tunnel: [_ w144 _] -> w77
          frame #0 {
            n271 = Wait (ms)(milliseconds to wait=u32 23000) -> ()  [unwired: 1 out]
          }
          frame #1 {
            n272 = while {
              tunnel: [w149] -> w145
              tunnel: [w148] -> w144
              stop <- w149 stop-if-true
              n273 = property on="21" class="Bool (strict)"() -> ("Top"=w147:i32)  [unwired: 2 in, 2 out]
              n274 = Add(x=w147, y=5) -> (x+y=w146:i32)
              n275 = Equal?(x=w146, y=215) -> (x = y?=w149:bool)
              n276 = property on="21" class="Bool (strict)"("Top"=w146) -> ()  [unwired: 2 in, 2 out]
              n277 = Wait Until Next ms Multiple(millisecond multiple=u32 50) -> ()  [unwired: 1 out]
              n278 = Tick Count (ms)() -> (millisecond timer value=w148:u32)
            }
          }
          frame #2 {
            n279 = property on="21" class="Bool (strict)"("Visible"=FALSE) -> ()  [unwired: 2 in, 2 out]
          }
        }
        n280 = stacked-sequence {
          tunnel: [_ w156 _] -> w54
          tunnel: [_ w155 _] -> w76
          frame #0 {
            n281 = Wait (ms)(milliseconds to wait=u32 24000) -> ()  [unwired: 1 out]
          }
          frame #1 {
            n282 = while {
              tunnel: [w160] -> w156
              tunnel: [w159] -> w155
              stop <- w160 stop-if-true
              n283 = property on="22" class="Bool (strict)"() -> ("Top"=w158:i32)  [unwired: 2 in, 2 out]
              n284 = Add(x=w158, y=5) -> (x+y=w157:i32)
              n285 = Equal?(x=w157, y=215) -> (x = y?=w160:bool)
              n286 = property on="22" class="Bool (strict)"("Top"=w157) -> ()  [unwired: 2 in, 2 out]
              n287 = Wait Until Next ms Multiple(millisecond multiple=u32 50) -> ()  [unwired: 1 out]
              n288 = Tick Count (ms)() -> (millisecond timer value=w159:u32)
            }
          }
          frame #2 {
            n289 = property on="22" class="Bool (strict)"("Visible"=FALSE) -> ()  [unwired: 2 in, 2 out]
          }
        }
        n290 = stacked-sequence {
          tunnel: [_ w167 _] -> w53
          tunnel: [_ w166 _] -> w75
          frame #0 {
            n291 = Wait (ms)(milliseconds to wait=u32 25000) -> ()  [unwired: 1 out]
          }
          frame #1 {
            n292 = while {
              tunnel: [w171] -> w167
              tunnel: [w170] -> w166
              stop <- w171 stop-if-true
              n293 = property on="23" class="Bool (strict)"() -> ("Top"=w169:i32)  [unwired: 2 in, 2 out]
              n294 = Add(x=w169, y=5) -> (x+y=w168:i32)
              n295 = Equal?(x=w168, y=215) -> (x = y?=w171:bool)
              n296 = property on="23" class="Bool (strict)"("Top"=w168) -> ()  [unwired: 2 in, 2 out]
              n297 = Wait Until Next ms Multiple(millisecond multiple=u32 50) -> ()  [unwired: 1 out]
              n298 = Tick Count (ms)() -> (millisecond timer value=w170:u32)
            }
          }
          frame #2 {
            n299 = property on="23" class="Bool (strict)"("Visible"=FALSE) -> ()  [unwired: 2 in, 2 out]
          }
        }
        n300 = stacked-sequence {
          tunnel: [_ w178 _] -> w52
          tunnel: [_ w177 _] -> w74
          frame #0 {
            n301 = Wait (ms)(milliseconds to wait=u32 26000) -> ()  [unwired: 1 out]
          }
          frame #1 {
            n302 = while {
              tunnel: [w182] -> w178
              tunnel: [w181] -> w177
              stop <- w182 stop-if-true
              n303 = property on="24" class="Bool (strict)"() -> ("Top"=w180:i32)  [unwired: 2 in, 2 out]
              n304 = Add(x=w180, y=5) -> (x+y=w179:i32)
              n305 = Equal?(x=w179, y=215) -> (x = y?=w182:bool)
              n306 = property on="24" class="Bool (strict)"("Top"=w179) -> ()  [unwired: 2 in, 2 out]
              n307 = Wait Until Next ms Multiple(millisecond multiple=u32 50) -> ()  [unwired: 1 out]
              n308 = Tick Count (ms)() -> (millisecond timer value=w181:u32)
            }
          }
          frame #2 {
            n309 = property on="24" class="Bool (strict)"("Visible"=FALSE) -> ()  [unwired: 2 in, 2 out]
            n310 = Wait Until Next ms Multiple(millisecond multiple=u32 1000) -> ()  [unwired: 1 out]
          }
        }
        n311 = Build Array(w79, w78, w77, w76, w75, w74) -> (w70:u32[])
        n312 = Compound Arithmetic op=AND(w57, w56, w55, w54, w53, w52) -> (w51:bool)
        n313 = Compound Arithmetic op=AND(w51, w50, w49, w48) -> (w46:bool)
        n314 = Build Array (concatenate)(w73, w72, w71, w70) -> (w47:u32[])
      }
      frame #2 {
        n315 = local read "press time"() -> (w494:u32[])
        n316 = Subtract(x=w494, y=w495) -> (x-y=w492:u32[])
        n317 = for {
          N: 24 -> [_]
          tunnel: w492 -> [w500] mode=indexing
          n318 = In Range and Coerce(upper limit=u32 300, x=w500, lower limit=u32 0) -> (In Range?=w497:bool)  [unwired: 1 out]
          n319 = case shown="True" w497 {
            frame False {
            }
            frame True {
              n320 = local read "score"() -> (w502:i32)
              n321 = Increment(x=w502) -> (x+1=w501:i32)
              n322 = local write "score"(w501) -> ()
            }
          }
        }
      }
      frame #3 {
        n323 = local read "score"() -> (w508:i32)
        n324 = while {
          tunnel: ["stop"] -> w503
          stop <- "stop" stop-if-true
        }
        n325 = Divide(x=w508, y=24) -> (x/y=w506:dbl)
        n326 = Multiply(x=w506, y=100.0) -> (x*y=→"Your Score":dbl)
      }
    }
  }
